vi "ICNC Move Arc XY Buf.vi"(0 "Sens":u32, 1 "Y_Target":i32, 2 "FAccelDecel":u32, 5 "I_Center":i32, 7 "J_Center":i32, 9 "X_Target":i32, 11 "error in (no error)":errorcluster caption="entrée d'erreur (pas d'erreur)", 12 "FStartStop":u32, 13 "Speed":u32) -> (4 "function return":u32, 15 "error out":errorcluster caption="sortie d'erreur")   [LabVIEW 2012, in "ICNC2.lvlib"]
doc: "DWORD ICNC_MoveArcXYBuf( DWORD Sens, int I_Center,\n int J_Center,\n int X_Target,\n int Y_Target,\n DWORD FStartStop,\n DWORD FAccelDecel,\n DWORD Speed);"
uses:
  <userlib>/ICNC/ICNC2.lvlib
  <userlib>/ICNC/ICNC2.dll
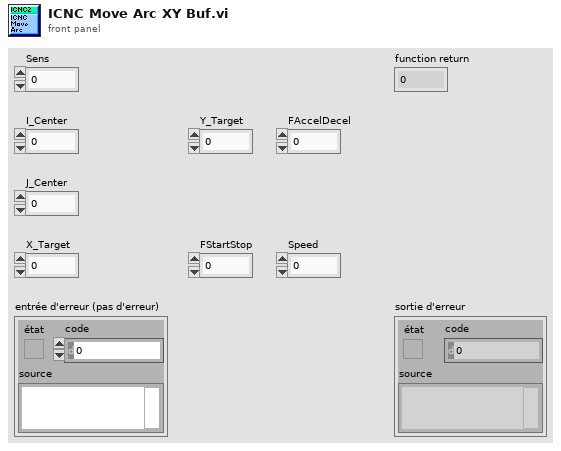
[diagram p1: front panel]
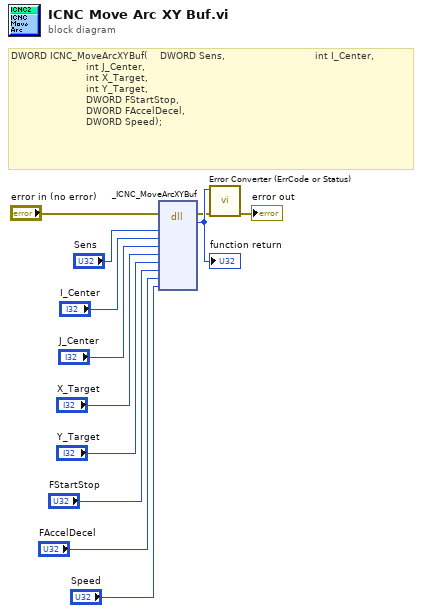
[diagram p0: block diagram]
diagram:
  # "DWORD ICNC_MoveArcXYBuf(    DWORD Sens,                              int I_Center,\n                         int J_Center,\n                         int X_Target,\n                         int Y_Target,\n                         DWORD FStartStop,\n                         DWORD FAccelDecel,\n                         DWORD Speed);"
  n1 = dll-call lib="C:/Program Files (x86)/National Instruments/LabVIEW 2012/user.lib/ICNC/ICNC2.*" fn="_ICNC_MoveArcXYBuf"(error in="error in (no error)", "Sens"="Sens", "I_Center"="I_Center", "J_Center"="J_Center", "X_Target"="X_Target", "Y_Target"="Y_Target", "FStartStop"="FStartStop", "FAccelDecel"="FAccelDecel", "Speed"="Speed") -> (error out=w2:errorcluster, w12:u32)  [unwired: 10 in, 1 out]
  "function return" <- w12
  n2 = call <userlib>:"Error Converter (ErrCode or Status).vi"("error in (no error)"=w2, "error code"=w12) -> ("error out"=→"error out":errorcluster)  [unwired: 9 in]
